vi "Generate Timestamped Filepath.vi"() -> ()   [LabVIEW 2019]
panel:
  out "Timestamped Filepath":path
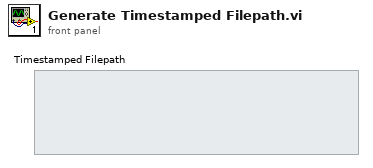
[diagram p1: front panel]
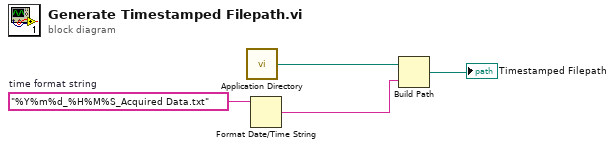
[diagram p0: block diagram]
diagram:
  w4 = "%Y%m%d_%H%M%S_Acquired Data.txt"  # time format string
  n1 = call <vilib>:"Application Directory.vi"() -> ("Application Directory"=w3:path)
  n2 = Format Date/Time String(time format string (%c)=w4) -> (date/time string=w2:string)  [unwired: 2 in]
  n3 = Build Path(base path=w3, name or relative path=w2) -> (appended path=→"Timestamped Filepath":path)
